vi "Beam Clock Mode Select.vi"(6 "Beam Clock Mode":enum8{"Trigger", "Toggle"}(ring)=enum."Toggle", 11 "Beam On":bool) -> (3 "Beam Clock Out":bool)   [LabVIEW 2014]
panel:
  # "Copyright 2014 Vidrio Technologies\nScanImage 5 software is licensed under the Apache License, Version 2.0 (the \"License\"); you may not use any files contained\nwithin the ScanImage 5 release except in compliance with the License. You may obtain a copy of the License at\n http://www.apache.org/licenses/LICENSE-2.0\nUnless required by applicable law or agreed to in writing, software distributed under the License is distributed on an\n\"AS IS\" BASIS, WITHOUT WARRANTIES OR CONDITIONS OF ANY KIND, either express or implied. See the License for the\n specific language governing permissions and limitations under the License."
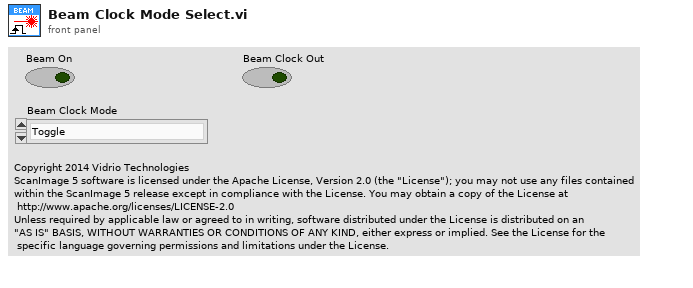
[diagram p1: front panel]
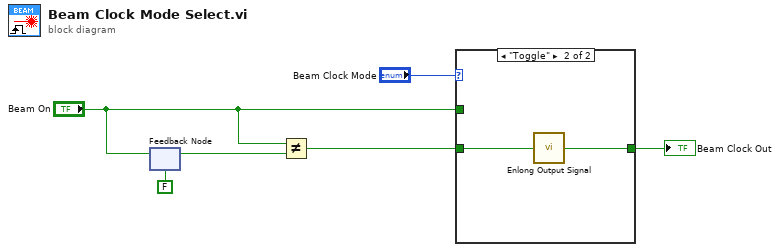
[diagram p0: block diagram]
diagram:
  n1 = feedback #1(FALSE) -> (w3:bool)
  n2 = feedback-in #1("Beam On") -> ()
  n3 = Not Equal?(x="Beam On", y=w3) -> (x != y?=w2:bool)
  n4 = case shown="\"Toggle\"" "Beam Clock Mode" {
    tunnel: "Beam On" -> [w7 _]
    tunnel: w2 -> [_ w8]
    tunnel: [w7 w9] -> w6
    frame "Trigger", Default {
    }
    frame "Toggle" {
      n5 = call "Enlong Output Signal.vi"("Trigger In"=w8) -> ("Trigger Out"=w9:bool)
    }
  }
  "Beam Clock Out" <- w6
